vi "Read Single Measurement (Voltage Harmonics).vi"(0 "VISA resource name":refnum<visa-resource-name>, 5 "Maximum Time (10000 ms)":i32=10000, 7 "Harmonic Order (1)":u8=1, 9 "Phase Order (1)":u8=1, 11 "error in (no error)":errorcluster) -> (3 "Total Voltage Harmonic Distortion":dbl, 4 "VISA resource name out":refnum<visa-resource-name>, 8 "Nth Voltage Harmonic Amplitude":dbl, 10 "Nth Voltage Harmonic Phase":dbl, 15 "error out":errorcluster)   [LabVIEW 2020, in "Agilent 681x Series.lvlib"]
doc: "Initiates the measurement and reads the selected order harmonic amplitude and phase values, and the voltage total harmonic distortion.\n\n<B>Note:</B>\n\nThis VI changes the <B>Trigger Source</B> to <B>Bus</B> and uses a software trigger after the instrument is initiated. If you want to control the triggering and other features, please use the low level VIs."
uses:
  <instrlib>/Agilent 681x Series/Agilent 681x Series.lvlib
  <instrlib>/Agilent 681x Series/Public/Data/Low Level/Fetch Single Measurement (Voltage Harmonics).vi
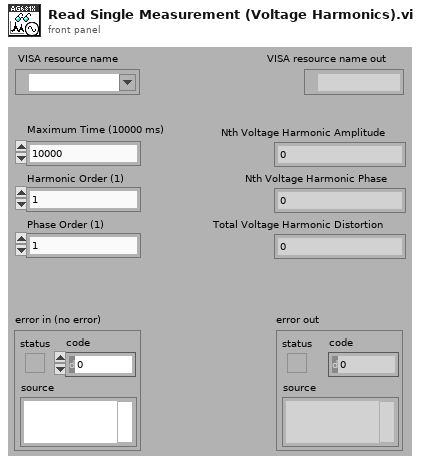
[diagram p1: front panel]
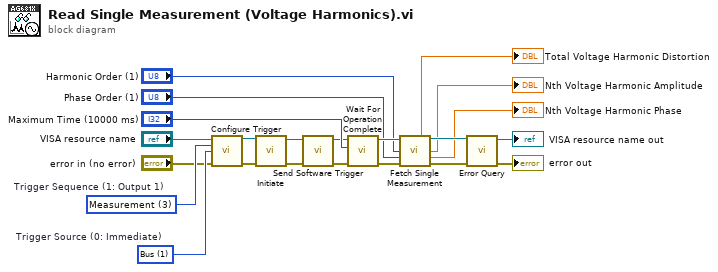
[diagram p0: block diagram]
diagram:
  w12 = 1 items=["Immediate", "Bus", "External", "Phase", "Trigger Out"]  # Trigger Source (0: Immediate)
  w13 = 3 items=["Output"=1, "Synchronous Source"=2, "Measurement"=3]  # Trigger Sequence (1: Output 1)
  n1 = call <instrlib>:"Configure Trigger.vi"("VISA resource name"="VISA resource name", "Trigger Sequence (1: Output 1)"=w13, "Trigger Source (0: Immediate)"=w12, "error in (no error)"="error in (no error)") -> ("VISA resource name out"=w10:refnum<visa-resource-name>, "error out"=w11:errorcluster)  [unwired: 10 in]
  n2 = call <instrlib>:"Initiate.vi"("error in (no error)"=w11, "VISA resource name"=w10) -> ("error out"=w9:errorcluster, "VISA resource name out"=w8:refnum<visa-resource-name>)  [unwired: 8 in]
  n3 = call <instrlib>:"Send Software Trigger.vi"("VISA resource name"=w8, "error in (no error)"=w9) -> ("VISA resource name out"=w6:refnum<visa-resource-name>, "error out"=w7:errorcluster)  [unwired: 12 in]
  n4 = call <instrlib>:"Wait For Operation Complete.vi"("error in (no error)"=w7, "Maximum Time (10000 ms)"="Maximum Time (10000 ms)", "VISA resource name"=w6) -> ("error out"=w21:errorcluster, "VISA resource name out"=w18:refnum<visa-resource-name>)  [unwired: 7 in]
  n5 = call-poly <instrlib>:"Fetch Single Measurement.vi"("VISA resource name"=w18, "Harmonic Order (1)"="Harmonic Order (1)", "Phase Order (1)"="Phase Order (1)", "error in (no error)"=w21) -> ("Total Voltage Harmonic Distortion"=→"Total Voltage Harmonic Distortion":dbl, "VISA resource name out"=w20:refnum<visa-resource-name>, "Nth Voltage Harmonic Amplitude"=→"Nth Voltage Harmonic Amplitude":dbl, "Nth Voltage Harmonic Phase"=→"Nth Voltage Harmonic Phase":dbl, "error out"=w19:errorcluster)  [unwired: 7 in]
  n6 = call <instrlib>:"Error Query.vi"("error in (no error)"=w19, "VISA resource name"=w20) -> ("error out"=→"error out":errorcluster, "VISA resource name out"=→"VISA resource name out":refnum<visa-resource-name>)  [unwired: 6 in, 2 out]
